vi "回文数质数2.vi"(3 "10的\n几次方":dbl) -> (0 "回文质数\n数量":dbl, 1 "回文质数":dbl[](array[numeric]))   [LabVIEW 2017]
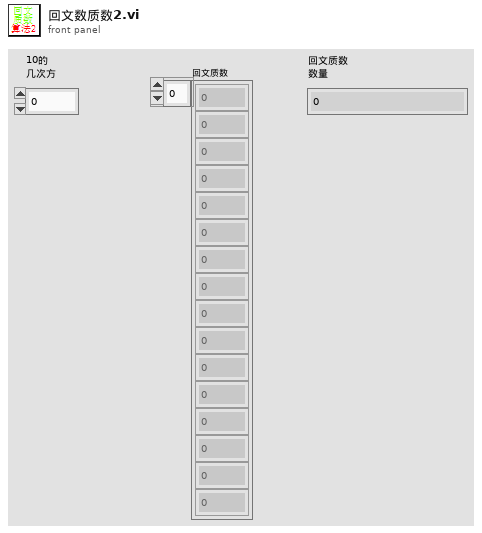
[diagram p1: front panel]
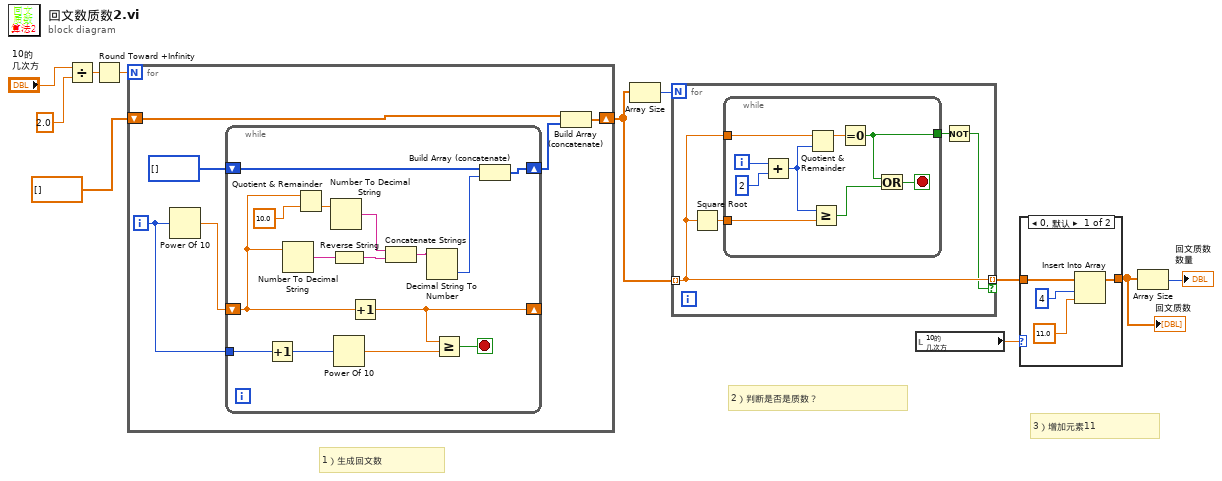
[diagram p0: block diagram]
diagram:
  # "3）增加元素11"
  # "2）判断是否是质数？"
  # "1）生成回文数"
  n1 = Divide(x="10的\n几次方", y=2.0) -> (x/y=w8:dbl)
  n2 = Round Toward +Infinity(x=w8) -> (ceil(x): smallest int >= x=w7:dbl)
  n3 = for {
    N: w7 -> [_]
    shift-right: [w16] -> w6
    shift-left: dbl[] [] -> [w17]
    i -> [w13]
    n4 = Power Of 10(x=w13) -> (10^x=w12:dbl)
    n5 = while {
      shift-right: [w28] -> _
      shift-left: w12 -> [w18]
      tunnel: w13 -> [w29]
      shift-right: [w31] -> w14
      shift-left: i32[] [] -> [w32]
      stop <- w26 stop-if-true
      n6 = Increment(x=w29) -> (x+1=w30:i32)
      n7 = Number To Decimal String(number=w18) -> (decimal integer string=w24:string)  [unwired: 1 in]
      n8 = Quotient & Remainder(x=w18, y=10.0) -> (floor(x/y)=w21:dbl)  [unwired: 1 out]
      n9 = Number To Decimal String(number=w21) -> (decimal integer string=w22:string)  [unwired: 1 in]
      n10 = Reverse String(1:w24) -> (0:w23:string)
      n11 = Power Of 10(x=w30) -> (10^x=w27:dbl)
      n12 = Increment(x=w18) -> (x+1=w28:dbl)
      n13 = Concatenate Strings(w22, w23) -> (w25:string)
      n14 = Decimal String To Number(string=w25) -> (number=w19:i32)  [unwired: 2 in, 1 out]
      n15 = Greater Or Equal?(x=w28, y=w27) -> (x >= y?=w26:bool)
      n16 = Build Array (concatenate)(w32, w19) -> (w31:i32[])
    }
    n17 = Build Array (concatenate)(w17, w14) -> (w16:dbl[])
  }
  n18 = Array Size(array=w6) -> (size(s)=w11:i32)
  n19 = for {
    N: w11 -> [_]
    tunnel: w6 -> [w34] mode=indexing
    tunnel: [w34] -> w3 mode=indexing if=w33
    n20 = Square Root(x=w34) -> (sqrt(x)=w36:dbl)
    n21 = while {
      tunnel: w36 -> [w41]
      tunnel: [w37] -> w35
      tunnel: w34 -> [w38]
      i -> [w44]
      stop <- w45 stop-if-true
      n22 = Add(x=w44, y=2) -> (x+y=w39:i32)
      n23 = Quotient & Remainder(x=w38, y=w39) -> (x-y*floor(x/y)=w42:dbl)  [unwired: 1 out]
      n24 = Greater Or Equal?(x=w39, y=w41) -> (x >= y?=w40:bool)
      n25 = Equal To 0?(x=w42) -> (x = 0?=w37:bool)
      n26 = Or(x=w37, y=w40) -> (x .or. y?=w45:bool)
    }
    n27 = Not(x=w35) -> (.not. x?=w33:bool)
  }
  n28 = local read "10的\n几次方"() -> (w4:dbl)
  n29 = case shown="0, 默认" w4 {
    tunnel: w3 -> [w47 w50]
    tunnel: [w46 w50] -> w1
    frame 0, Default {
      n30 = Insert Into Array(array=w47, index=4 ("索引"), new element=11.0 ("新元素/子数组")) -> (w46:dbl[])
    }
    frame 1 {
    }
  }
  "回文质数" <- w1
  n31 = Array Size(array=w1) -> (size(s)=→"回文质数\n数量":i32)
